vi "Get Mode.vi"(8 "error in (no error)":errorcluster, 11 "Stream in":refnum<class "Stream.lvclass">) -> (0 "error out":errorcluster, 2 "Mode":T1, 3 "Stream out":refnum<class "Stream.lvclass">)   [LabVIEW 2020, in "Stream.lvlib" / "Stream.lvclass"]
uses:
  Stream.lvclass
  Mode.ctl
  Stream.lvclass/Stream.ctl
  Stream.lvlib
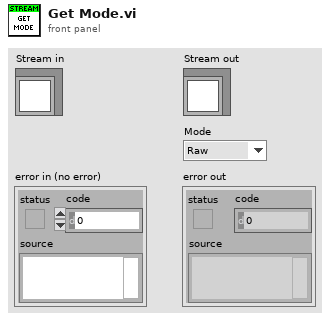
[diagram p1: front panel]
types:
  T1 = typedef "Stream.lvlib/Mode.ctl" = enum16{"Raw", "Buffered", "LineTerm"}
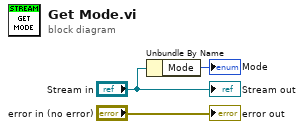
[diagram p0: block diagram]
diagram:
  n1 = Unbundle By Name("Stream in") -> ("Mode"=→"Mode":T1)
  "error out" <- "error in (no error)"
  "Stream out" <- "Stream in"
